vi "1.3.2-Serial Write.vi"(0 "Tx FPGA I/O":refnum<k21>="Tx", 1 "Write FIFO":refnum<k21>="Write FIFO", 7 "baud rate (9600)":u32=9600, 9 "data bits (8)":i32=8 min=5 max=8 step=1, 11 "parity (0:none)":enum16{"None", "Odd", "Even", "Mark", "Space"}(ring), 12 "stop bits (10: 1 bit)":u16(ring)=10 items=["1.0"=10, "1.5"=15, "2.0"=20], 13 "Invert Polarity?":bool) -> ()   [LabVIEW 2010]
uses:
  <vilib>/eio/EIONode/EIONode.xnode
  <vilib>/rvi/eio/nirviEIOImplementation/nirviEIOImplementation.xnode
  <vilib>/rvi/eio/common/nirviEmuClasses.ctl
  <vilib>/rvi/DataTransferAndStorage/Container/XNode/niFpgaContainer.xnode
  <vilib>/rvi/DataTransferAndStorage/Container/Common/niFpgaTransferTypeControl.ctl
  <vilib>/rvi/FIFO/Fifo_Types/niFpgaFifoControlLogicControl.ctl
  <vilib>/rvi/DataTransferAndStorage/Container/Common/niFpgaContainerMethod.ctl
  <vilib>/rvi/DataTransferAndStorage/Container/Common/niFpgaContainerMetaDataKey.ctl
  <vilib>/rvi/DataTransferAndStorage/FIFO/niFpgaPeerToPeerStreamState.ctl
  <vilib>/rvi/eio/common/nirviEmuTemplateMethod_noerrors.vi
  1.0-Hindbrain Global.vi
  <vilib>/rvi/DataTransferAndStorage/Container/Common/niFpgaContainerExecOnDevCompGetState.vi
  <vilib>/rvi/FIFO/Fifo_Resource/nirvififoEmulationSetSize.vi
  <vilib>/rvi/DataTransferAndStorage/Container/Common/niFpgaContainerGetUniqueNameForEmu.vi
  <vilib>/rvi/interface/RandomDataEmulation/nirviRandomDataFPGAFIFO.vi
  <vilib>/rvi/interface/RandomDataEmulation/niFpgaRandomDataHandleErrors.vi
  <vilib>/rvi/eio/common/nirviEmuReportErrorAndStop.vi
panel:
  out "Read: Transmission Error":bool
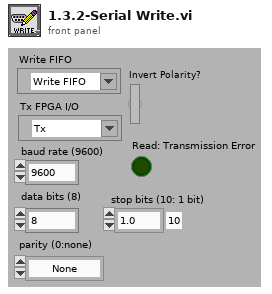
[diagram p1: front panel]
types:
  T1 = typedef "nirviEmuClasses.ctl" = enum16{"IO Read", "IO Write", "Method", "Property Read", "Property Write"}
  T2 = typedef "niFpgaFifoControlLogicControl.ctl" = enum16{"Slice Fabric", "Target Optimal", "Built-in"}
  T3 = typedef "niFpgaContainerMethod.ctl" = enum16{"<none>", "write", "read", "clear", "getNumberOfElementsToWrite", "getNumberOfElementsToRead", "enable", "disable", "flushAndDisable", "getStreamState", "readA", "readB", "dramWrite", "dramWriteWithByteEnables", "dramRequestData", "dramRetrieveData"}
  T4 = typedef "niFpgaTransferTypeControl.ctl" = enum16{"Target-Scoped", "Host to Target - DMA", "Target to Host - DMA", "Peer to Peer Reader", "Peer to Peer Writer", "Bidirectional"}
  T5 = typedef "niFpgaPeerToPeerStreamState.ctl" = enum16{"Unlinked", "Disabled", "Enabled", "Flushing"}
  T6 = typedef "niFpgaContainerMetaDataKey.ctl" = enum16{"FPGA FIFO", "FPGA Memory", "FPGA Register"}
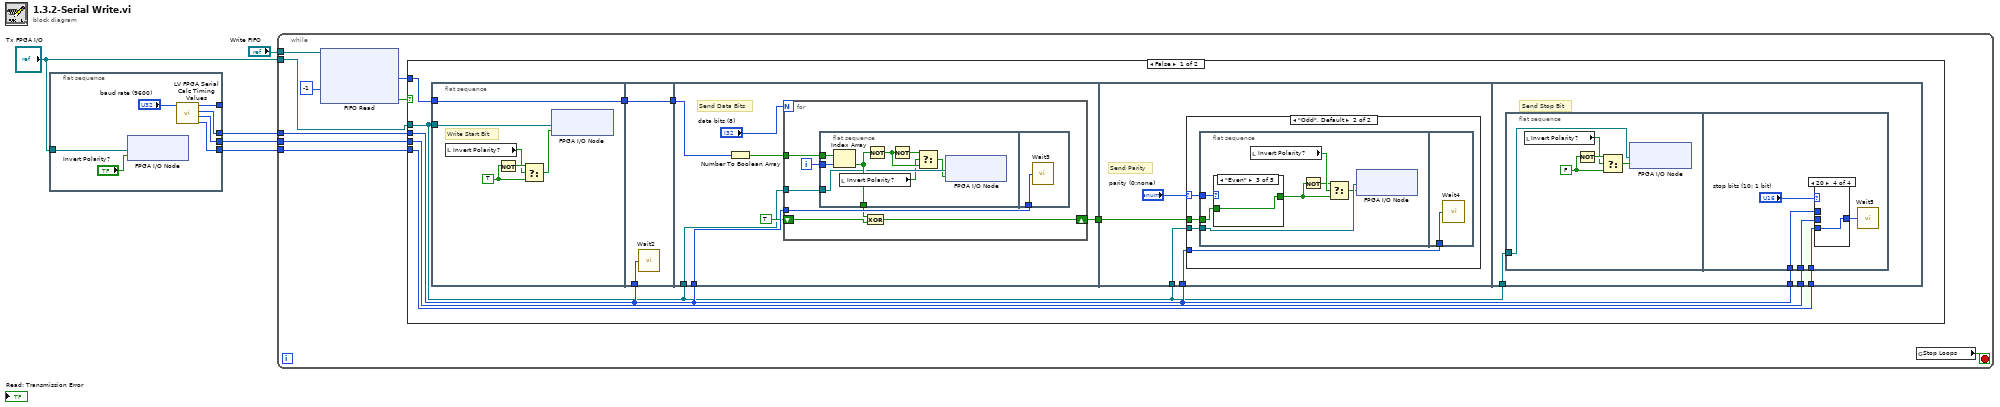
[diagram p0: block diagram]
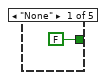
[diagram p3: hidden frame]
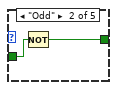
[diagram p4: hidden frame]
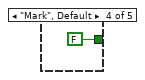
[diagram p5: hidden frame]
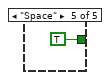
[diagram p6: hidden frame]
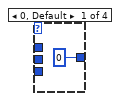
[diagram p7: hidden frame]
diagram:
  n1 = flat-sequence {
    tunnel: [w8] -> w5
    tunnel: [w11] -> _
    tunnel: [w10] -> w4
    tunnel: [w9] -> w3
    tunnel: "Tx FPGA I/O" -> [w7]
    frame #0 {
      n2 = xnode "FPGA I/O Node"("I/O Item"="Invert Polarity?", "FPGA I/O In"=w7) -> ()  [unwired: 1 out]
      n3 = call "LV FPGA Serial Calc Timing Values.vi"("baud rate (1000000)"="baud rate (9600)") -> ("Two Bit"=w9:u32, "One and Half Bit"=w10:u32, "One Bit"=w8:u32, "Half Bit"=w11:u32)  [unwired: 1 in, 2 out]
    }
  }
  n4 = while {
    tunnel: w3 -> [w32]
    tunnel: w4 -> [w31]
    tunnel: w5 -> [w30]
    tunnel: "Tx FPGA I/O" -> [w29]
    tunnel: "Write FIFO" -> [w25]
    stop <- w24 stop-if-true
    n5 = xnode ("FIFO Read")("Timeout"=-1, "FIFO In"=w25) -> ("Element"=w28:u8, "Timed Out?"=w26:bool)  [unwired: 1 out]
    n6 = case shown="False" w26 {
      tunnel: w32 -> [w354 _]
      tunnel: w31 -> [w353 _]
      tunnel: w30 -> [w352 _]
      tunnel: w29 -> [w351 _]
      tunnel: w28 -> [w350 _]
      frame False {
        n7 = flat-sequence {
          tunnel: w351 -> [w363]
          tunnel: w350 -> [w358]
          tunnel: [w358] -> w357
          tunnel: w352 -> [w376]
          tunnel: [w375] -> w356
          tunnel: w357 -> [w375]
          tunnel: w352 -> [w383]
          tunnel: [w381] -> w355
          tunnel: w351 -> [w379]
          tunnel: w356 -> [w378]
          tunnel: w352 -> [w413]
          tunnel: w355 -> [w414]
          tunnel: w351 -> [w412]
          tunnel: w352 -> [w447]
          tunnel: w353 -> [w446]
          tunnel: w354 -> [w445]
          tunnel: w351 -> [w444]
          frame #0 {
            w361 = TRUE
            # "Write Start Bit"
            n8 = local read "Invert Polarity?"() -> (w360:bool)
            n9 = Not(x=w361) -> (.not. x?=w362:bool)
            n10 = Select(t=w362, s=w360, f=w361) -> (s? t:f=w359:bool)
            n11 = xnode "FPGA I/O Node"("I/O Item"=w359, "FPGA I/O In"=w363) -> ()  [unwired: 1 out]
          }
          frame #1 {
            n12 = call "Wait2"("Count(Ticks)"=w376) -> ()  [unwired: 1 out]
          }
          frame #2 {
            # "Send Data Bits"
            n13 = Number To Boolean Array(number=w378) -> (Boolean array=w380:bool[])
            n14 = for {
              N: "data bits (8)" -> [_]
              tunnel: w383 -> [w387]
              shift-right: [w390] -> w381
              shift-left: TRUE -> [w389]
              tunnel: w380 -> [w386]
              tunnel: w379 -> [w384]
              i -> [w388]
              n15 = flat-sequence {
                tunnel: w388 -> [w398]
                tunnel: w386 -> [w397]
                tunnel: [w396] -> w385
                tunnel: w384 -> [w395]
                tunnel: w387 -> [w410]
                frame #0 {
                  n16 = Index Array(array=w397, index=w398) -> (element=w396:bool)
                  n17 = local read "Invert Polarity?"() -> (w392:bool)
                  n18 = Not(x=w396) -> (.not. x?=w393:bool)
                  n19 = Not(x=w393) -> (.not. x?=w394:bool)
                  n20 = Select(t=w394, s=w392, f=w393) -> (s? t:f=w391:bool)
                  n21 = xnode "FPGA I/O Node"("I/O Item"=w391, "FPGA I/O In"=w395) -> ()  [unwired: 1 out]
                }
                frame #1 {
                  n22 = call "Wait3"("Count(Ticks)"=w410) -> ()  [unwired: 1 out]
                }
              }
              n23 = Exclusive Or(1:w389, 2:w385) -> (0:w390:bool)
            }
          }
          frame #3 {
            # "Send Parity"
            n24 = case shown="\"Odd\", Default" "parity (0:none)" {
              selector: "parity (0:none)" -> [_ w418]
              tunnel: w414 -> [_ w417]
              tunnel: w413 -> [_ w416]
              tunnel: w412 -> [_ w415]
              frame "None" {
              }
              frame "Odd", Default {
                n25 = flat-sequence {
                  tunnel: w417 -> [w424]
                  tunnel: w418 -> [w425]
                  tunnel: w415 -> [w423]
                  tunnel: w416 -> [w443]
                  frame #0 {
                    n26 = case shown="\"Even\"" w425 {
                      tunnel: w424 -> [_ w439 w440 _ _]
                      tunnel: [FALSE ("y") w438 w440 FALSE ("y") TRUE ("y")] -> w420
                      frame "None" {
                      }
                      frame "Odd" {
                        n27 = Not(x=w439) -> (.not. x?=w438:bool)
                      }
                      frame "Even" {
                      }
                      frame "Mark", Default {
                      }
                      frame "Space" {
                      }
                    }
                    n28 = local read "Invert Polarity?"() -> (w422:bool)
                    n29 = Not(x=w420) -> (.not. x?=w421:bool)
                    n30 = Select(t=w421, s=w422, f=w420) -> (s? t:f=w419:bool)
                    n31 = xnode "FPGA I/O Node"("I/O Item"=w419, "FPGA I/O In"=w423) -> ()  [unwired: 1 out]
                  }
                  frame #1 {
                    n32 = call "Wait4"("Count(Ticks)"=w443) -> ()  [unwired: 1 out]
                  }
                }
              }
            }
          }
          frame #4 {
            # "Send Stop Bit"
            n33 = flat-sequence {
              tunnel: w444 -> [w452]
              tunnel: w447 -> [w468]
              tunnel: w446 -> [w467]
              tunnel: w445 -> [w466]
              frame #0 {
                w450 = FALSE
                n34 = local read "Invert Polarity?"() -> (w449:bool)
                n35 = Not(x=w450) -> (.not. x?=w451:bool)
                n36 = Select(t=w451, s=w449, f=w450) -> (s? t:f=w448:bool)
                n37 = xnode "FPGA I/O Node"("I/O Item"=w448, "FPGA I/O In"=w452) -> ()  [unwired: 1 out]
              }
              frame #1 {
                n38 = case shown="20" "stop bits (10: 1 bit)" {
                  tunnel: w468 -> [_ w470 _ _]
                  tunnel: w467 -> [_ _ w471 _]
                  tunnel: w466 -> [_ _ _ w472]
                  tunnel: [u32 0 ("One Bit") w470 w471 w472] -> w465
                  frame 0, Default {
                  }
                  frame 10 {
                  }
                  frame 15 {
                  }
                  frame 20 {
                  }
                }
                n39 = call "Wait5"("Count(Ticks)"=w465) -> ()  [unwired: 1 out]
              }
            }
          }
        }
      }
      frame True {
      }
    }
    n40 = global read "1.0-Hindbrain Global.vi" "Stop Loops"() -> (w24:bool)
  }
